vi "Project Initializer - Clear _Source Folder.vi"(8 "error in (no error)":errorcluster, 10 "Source Project Name":string, 11 "Project _Source Directory":path) -> (0 "error out":errorcluster)   [LabVIEW 2022 SP3]
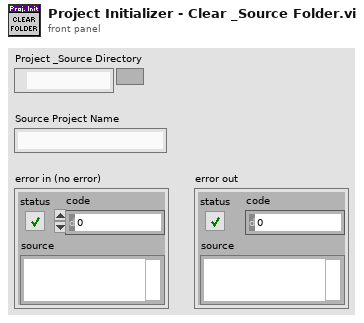
[diagram p1: front panel]
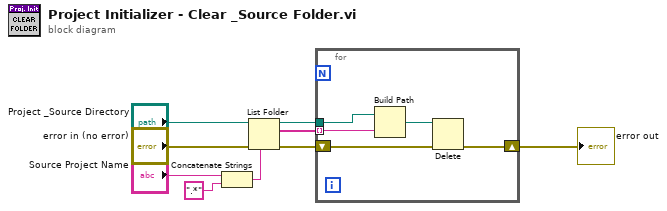
[diagram p0: block diagram]
diagram:
  n1 = Concatenate Strings("Source Project Name", ".*" ("string")) -> (w2:string)
  n2 = List Folder(path="Project _Source Directory", pattern=w2, error in="error in (no error)") -> (path out=w5:path, filenames=w4:string[], error out=w6:errorcluster)  [unwired: 1 in, 1 out]
  n3 = for {
    tunnel: w4 -> [w12] mode=indexing
    tunnel: w5 -> [w14]
    shift-right: [w10] -> w9
    shift-left: w6 -> [w11]
    n4 = Build Path(base path=w14, name or relative path=w12) -> (appended path=w13:path)
    n5 = Delete(path (use dialog)=w13, error in=w11) -> (error out=w10:errorcluster)  [unwired: 3 in, 2 out]
  }
  "error out" <- w9
